vi "while.vi"() -> ()   [LabVIEW 2017]
panel:
  in  "停止":bool
  out "布尔":bool
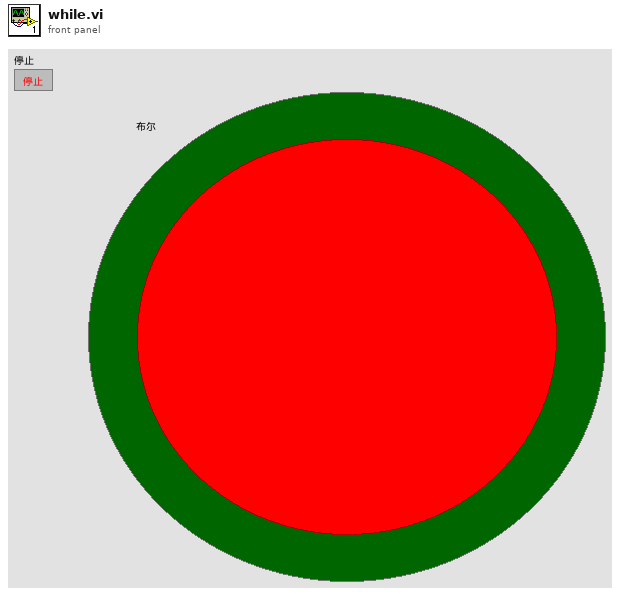
[diagram p1: front panel]
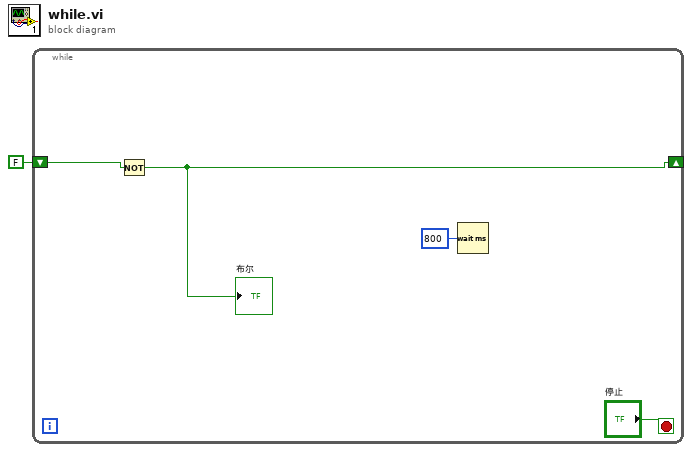
[diagram p0: block diagram]
diagram:
  n1 = while {
    shift-right: [w3] -> _
    shift-left: FALSE -> [w4]
    stop <- "停止" stop-if-true
    n2 = Not(x=w4) -> (.not. x?=w3:bool)
    "布尔" <- w3
    n3 = Wait (ms)(milliseconds to wait=u32 800 ("等待时间（毫秒）")) -> ()  [unwired: 1 out]
  }
